vi "Begin.vi"(8 "error in":errorcluster) -> (0 "error out":errorcluster)   [LabVIEW 2020]
doc: "Called before other user functions, this VI is expected to open initial I/O refnums, load in file data, and do all program initialization. Notice that the <B>error out</B> terminal is simply used for data flow. Wiring it to other structures or subVIs ensures that this VI runs first."
uses:
  <vilib>/Rock Robotics/WPI/ThirdParty/Phoenix-LabVIEW/Pigeon2/controls/CTRE_Phoenix_Pigeon2_Configurables.ctl
  <vilib>/Rock Robotics/WPI/DriverStation/WPI_DriverStationRobotMode2.ctl
  <vilib>/Rock Robotics/SystemInterfaces/i2clib/i2c_bus.ctl
  <vilib>/Rock Robotics/WPI/Solenoid/WPI_SolenoidChannel.ctl
  <vilib>/Rock Robotics/SystemInterfaces/DIO/FPGA_DIOChannel.ctl
  <vilib>/Rock Robotics/WPI/Joystick/WPI_JoystickDeviceEnum.ctl
  Robot Global Data.vi
  <vilib>/Rock Robotics/WPI/Solenoid/WPI_SolenoidOpenDouble.vi
  <vilib>/Rock Robotics/WPI/Utilities/WPI_GetSetVariantRefNum.vi
  <vilib>/Rock Robotics/WPI/Switch/WPI_SwitchOpenCounting.vi
  <vilib>/Rock Robotics/WPI/Switch/WPI_SwitchOpenLimit.vi
  <vilib>/Rock Robotics/WPI/ThirdParty/Phoenix-LabVIEW/Motor Controller/Get/CTRE_Phoenix_MotorController_GetSelectedSensorData.vi
panel:
  in  "Pigeon2 Configurables":T1
  # "Yaw Angle needed to reach the current orientation in degrees"
  # "Configures the mounting pose of the Pigeon2\nThis is the yaw-pitch-roll teh Pigeon2 underwent to get to its current orientation,\n referenced from the robot's point of view\nThis is only necessary if the Pigeon2 is mounted at an exotic angle near the gimbal lock point or not forward.\nIf the pigeon is relatively flat and pointed forward, this is not needed"
  # "Pitch Angle needed to reach the current orientation in degrees"
  # "Roll Angle needed to reach the current orientation in degrees"
  # "Disables the temperature compensation\nfrom the Pigeon2. It is recommended that\nthis remains false"
  # "Disables the no-motion calibration from the\nPigeon2. It is recommended that this \nremains false"
  # "Enables the compass for Pigeon2\nThis is not recommended for any indoor robotics"
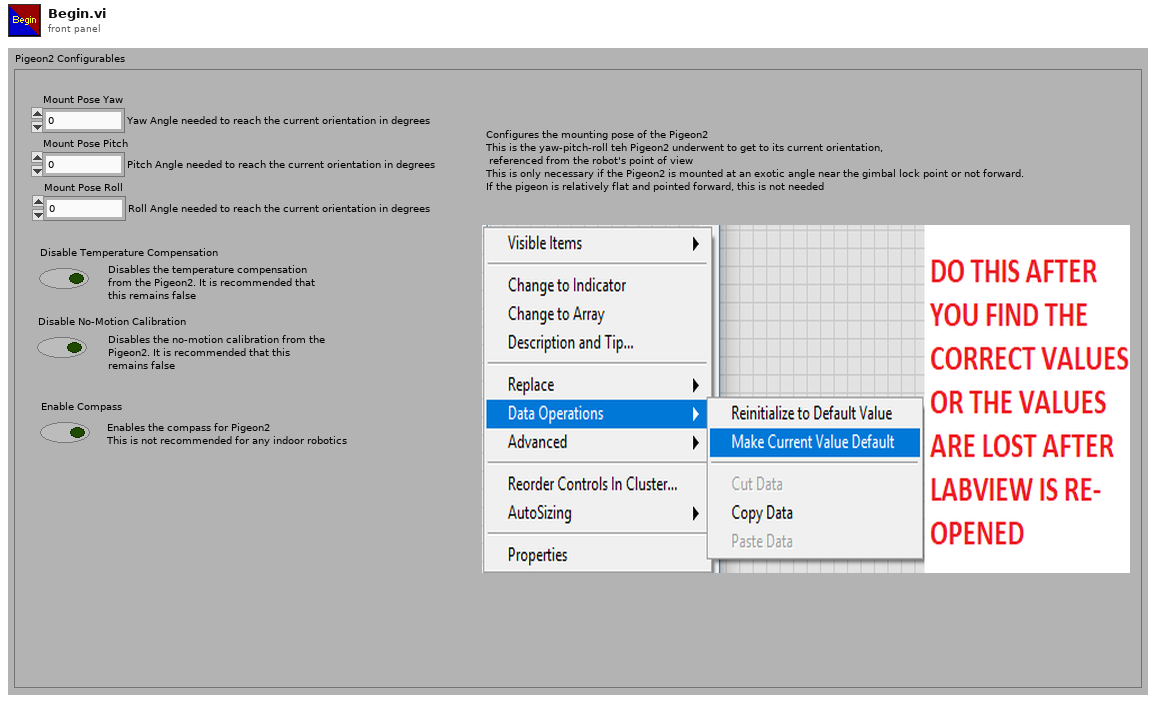
[diagram p1: front panel]
types:
  T1 = typedef "CTRE_Phoenix_Pigeon2_Configurables.ctl" = cluster{"Mount Pose Yaw":dbl, "Mount Pose Pitch":dbl, "Mount Pose Roll":dbl, "Disable Temperature Compensation":bool, "Disable No-Motion Calibration":bool, "Enable Compass":bool}
  T2 = typedef "FPGA_DIOChannel.ctl" = enum8{"DIO 0", "DIO 1", "DIO 2", "DIO 3", "DIO 4", "DIO 5", "DIO 6", "DIO 7", "DIO 8", "DIO 9", "DIO MXP 0", "DIO MXP 1", "DIO MXP 2", "DIO MXP 3", "DIO MXP 4", "DIO MXP 5", "DIO MXP 6", "DIO MXP 7", "DIO MXP 8", "DIO MXP 9", "DIO MXP 10", "DIO MXP 11", "DIO MXP 12", "DIO MXP 13", "DIO MXP 14", "DIO MXP 15", "SPI Port CS1", "SPI Port CS2", "SPI Port CS3", "SPI Port MISO", "SPI Port MOSI", "Invalid"}
  T3 = typedef "WPI_JoystickDeviceEnum.ctl" = enum16{"USB 0", "USB 1", "USB 2", "USB 3", "USB 4", "USB 5"}
  T4 = typedef "WPI_SolenoidChannel.ctl" = enum8{"Solenoid 0", "Solenoid 1", "Solenoid 2", "Solenoid 3", "Solenoid 4", "Solenoid 5", "Solenoid 6", "Solenoid 7", "Solenoid 8", "Solenoid 9", "Solenoid 10", "Solenoid 11", "Solenoid 12", "Solenoid 13", "Solenoid 14", "Solenoid 15", "Invalid"}
  T5 = typedef "i2c_bus.ctl" = enum16{"I2C On-Board", "I2C MXP", "Invalid"}
  T6 = typedef "WPI_DriverStationRobotMode2.ctl" = enum16{"Autonomous Disabled", "Autonomous Enabled", "Teleop Disabled", "Teleop Enabled", "Disconnected", "Finish", "Test Disabled", "Test Enabled", "Emergency Stopped"}
  T7 = typedef "WPI_JoystickDevRef.ctl" = cluster{"Device":T3}
  T8 = typedef "WPI_CompressorDevRef.ctl" = cluster{"DevStatus":errorcluster, "Pneumatics Control Module":u8}
  T9 = typedef "Color Sensor V3 DevRef.ctl" = cluster{"I2CDevRef":T10}
  T10 = typedef "WPI_I2CDevRef.ctl" = cluster{"DevStatus":errorcluster, "Device Address":u8, "Handle":i32, "I2C Bus":T5}
  T11 = typedef "WPI_SolenoidDevRef.ctl" = cluster{"DevStatus":errorcluster, "Pneumatics Control Module":u8, "Forward Solenoid Channel":T4, "Reverse Solenoid Channel":T4}
  T12 = typedef "WPI_MotorControlDeviceRef.ctl" = cluster{"DeviceStatus":errorcluster, "Type":T13, "PWM":cluster{"PWM Channel":T14, "DeadBand":T15}, "CAN":cluster{"Device Number":u8, "SetOutput VI Ref":variant, "GetOutput VI Ref":variant, "Enable VI Ref":variant, "Disable VI Ref":variant, "Data":variant}, "Invert":bool, "DIO PWM":cluster{"PWM \"Enable\" Channel":T14, "DIOChannel":T2, "PWM Rate":dbl}}
  T13 = typedef "WPI_MotorControlType.ctl" = enum16{"PWM", "CAN", "DIO PWM"}
  T14 = typedef "FPGA_DIOPWMChannel.ctl" = enum8{"PWM 0", "PWM 1", "PWM 2", "PWM 3", "PWM 4", "PWM 5", "PWM 6", "PWM 7", "PWM 8", "PWM 9", "PWM MXP 0", "PWM MXP 1", "PWM MXP 2", "PWM MXP 3", "PWM MXP 4", "PWM MXP 5", "PWM MXP 6", "PWM MXP 7", "PWM MXP 8", "PWM MXP 9", "Invalid"}
  T15 = typedef "WPI_PWMDeadband.ctl" = cluster{"Name":string, "maxPositivePwm":i32, "minPositivePwm":i32, "centerPwm":i32, "maxNegativePwm":i32, "minNegativePwm":i32, "angularRange":u16}
  T16 = typedef "CTRE_PigeonIMU_DeviceRef.ctl" = cluster{"DeviceStatus":errorcluster, "Device Number":u8, "Type":T17, "Device ID":u32, "Handle":u64, "UsageFrame":u32, "Library Path":path}
  T17 = typedef "CTRE_PigeonIMU_ConnectionType.ctl" = u32
  T18 = typedef "CTRE_Phoenix_CANcoder_DeviceRef.ctl" = cluster{"DeviceStatus":errorcluster, "Device Number":u8, "Handle":u64, "UsageFrame":u32, "Library Path":path}
  T19 = typedef "WPI_SwitchDevRef.ctl" = cluster{"DevStatus":errorcluster, "DIO Channel":T2, "CntIndex":T20, "Normally Closed":bool}
  T20 = typedef "FPGA_CounterCtrSystemIndex.ctl" = enum8{"Ctr 0", "Ctr 1", "Ctr 2", "Ctr 3", "Ctr 4", "Ctr 5", "Ctr 6", "Ctr 7", "Invalid"}
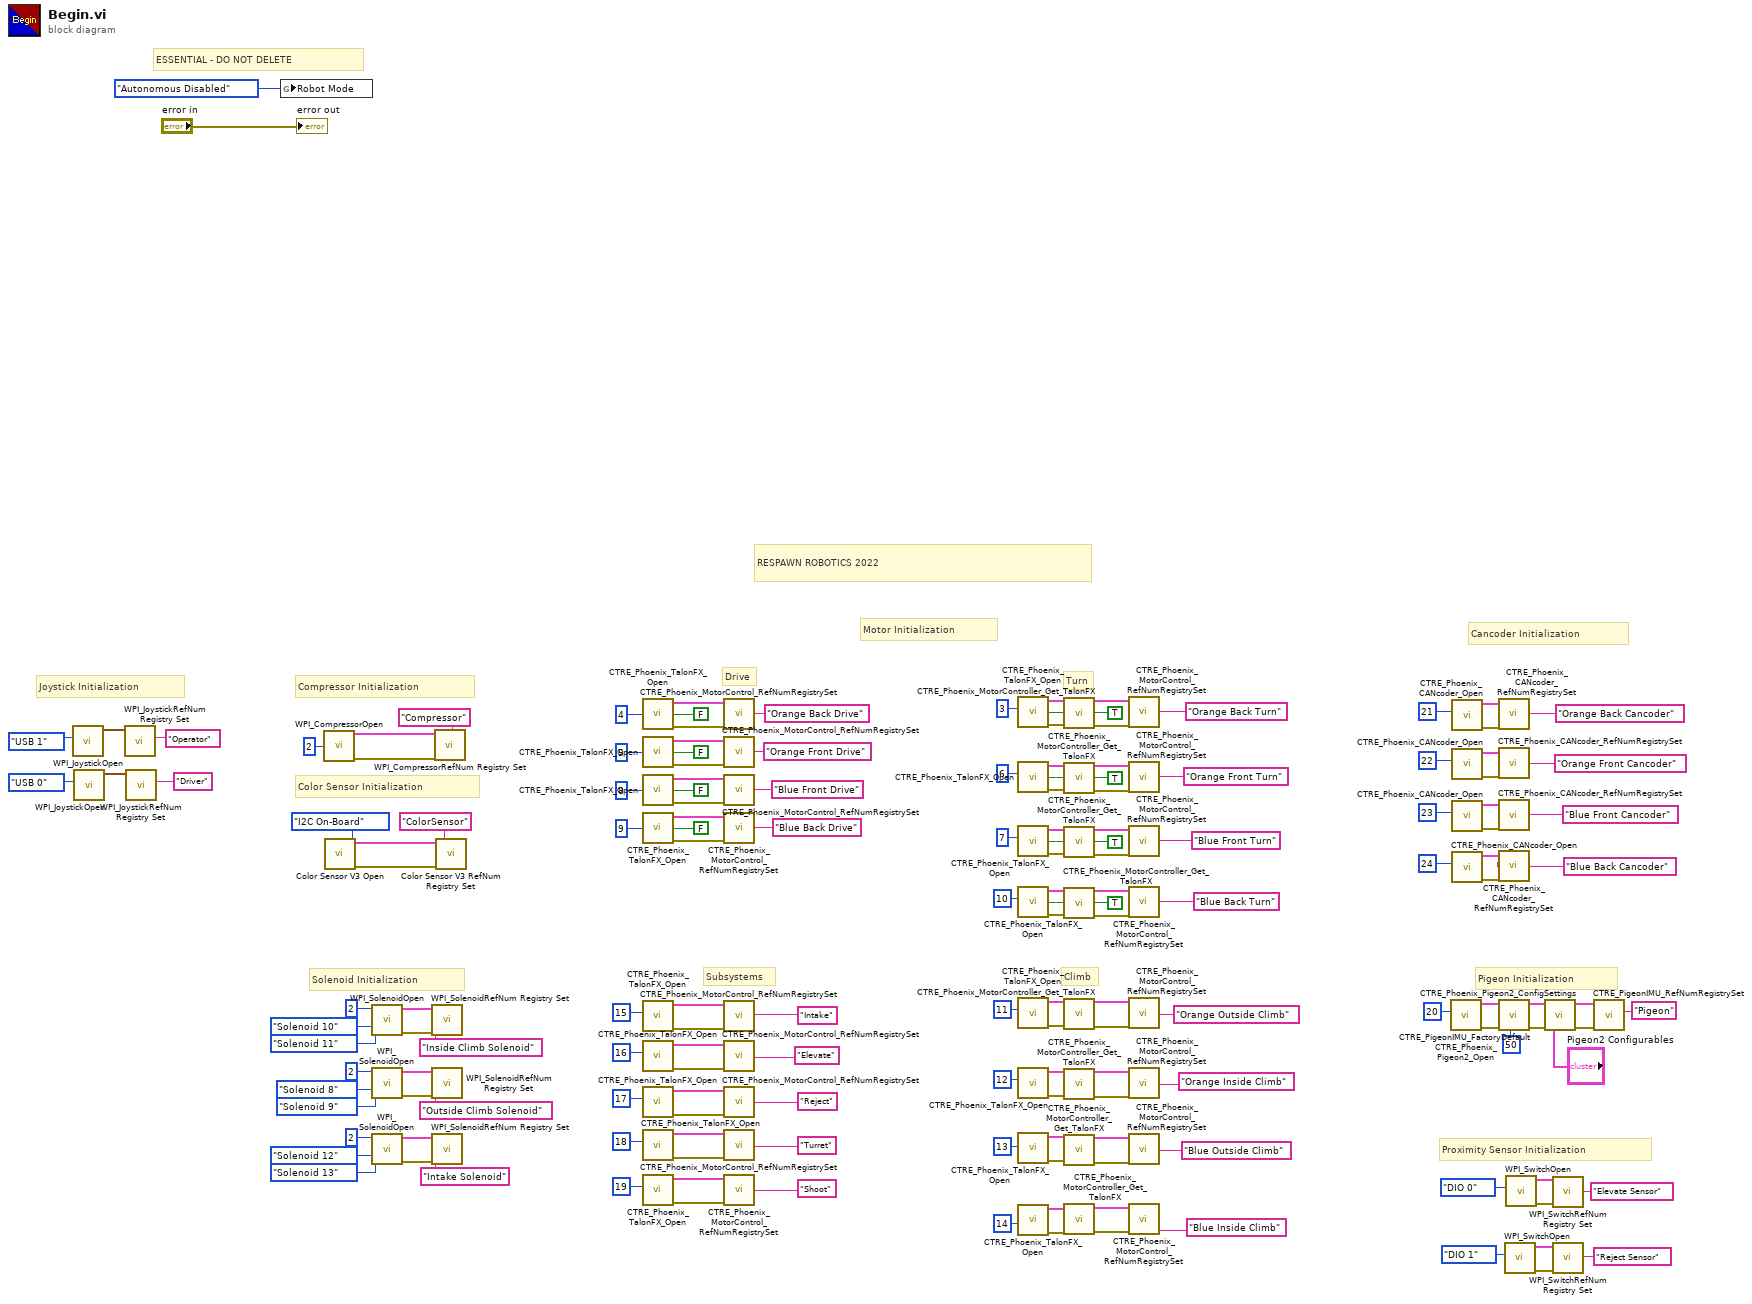
[diagram p0: block diagram]
diagram:
  # "Proximity Sensor Initialization"
  # "Pigeon Initialization"
  # "Cancoder Initialization"
  # "Solenoid Initialization"
  # "Color Sensor Initialization"
  # "Compressor Initialization"
  # "Climb"
  # "Subsystems"
  # "Turn"
  # "Drive"
  # "Motor Initialization"
  # "Joystick Initialization"
  # "RESPAWN ROBOTICS 2022"
  # "ESSENTIAL - DO NOT DELETE"
  n1 = call <vilib>:"WPI_JoystickOpen.vi"("JoystickDevice"=WPI_JoystickDeviceEnum."USB 1") -> ("JoystickDevRef"=w118:T7)  [unwired: 10 in]
  n2 = call <vilib>:"WPI_JoystickOpen.vi"("JoystickDevice"=WPI_JoystickDeviceEnum."USB 0") -> ("JoystickDevRef"=w121:T7)  [unwired: 10 in]
  n3 = call <vilib>:"WPI_JoystickRefNum Registry Set.vi"("refnum name"="Operator", "JoystickDevRef"=w118) -> ()  [unwired: 8 in, 2 out]
  n4 = call <vilib>:"WPI_JoystickRefNum Registry Set.vi"("refnum name"="Driver", "JoystickDevRef"=w121) -> ()  [unwired: 8 in, 2 out]
  n5 = global write "Robot Global Data.vi" "Robot Mode"(WPI_DriverStationRobotMode2."Autonomous Disabled" ("Robot Mode")) -> ()
  n6 = call <vilib>:"WPI_CompressorOpen.vi"("Pneumatics device (def)"=u8 2) -> ("CompressorDevRef"=w151:T8, "error out"=w152:errorcluster)  [unwired: 13 in]
  n7 = call <vilib>:"Color Sensor V3 Open.vi"("I2C Bus"=i2c_bus."I2C On-Board") -> ("error out"=w158:errorcluster, "ColorSensorDevRef"=w157:T9)  [unwired: 9 in]
  n8 = call-poly <vilib>:"WPI_SolenoidOpen.vi"("Reverse Solenoid Channel"=WPI_SolenoidChannel."Solenoid 11", "Forward Solenoid Channel"=WPI_SolenoidChannel."Solenoid 10", "Pneumatics Device (def)"=u8 2) -> ("error out"=w154:errorcluster, "SolenoidDevRef"=w153:T11)  [unwired: 7 in]
  n9 = call-poly <vilib>:"WPI_SolenoidOpen.vi"("Reverse Solenoid Channel"=WPI_SolenoidChannel."Solenoid 9", "Forward Solenoid Channel"=WPI_SolenoidChannel."Solenoid 8", "Pneumatics Device (def)"=u8 2) -> ("error out"=w140:errorcluster, "SolenoidDevRef"=w139:T11)  [unwired: 7 in]
  n10 = call-poly <vilib>:"WPI_SolenoidOpen.vi"("Reverse Solenoid Channel"=WPI_SolenoidChannel."Solenoid 13", "Forward Solenoid Channel"=WPI_SolenoidChannel."Solenoid 12", "Pneumatics Device (def)"=u8 2) -> ("error out"=w138:errorcluster, "SolenoidDevRef"=w137:T11)  [unwired: 7 in]
  n11 = call <vilib>:"WPI_SolenoidRefNum Registry Set.vi"("error in (no error)"=w154, "refnum name"="Inside Climb Solenoid", "SolenoidDevRef"=w153) -> ()  [unwired: 7 in, 2 out]
  n12 = call <vilib>:"WPI_SolenoidRefNum Registry Set.vi"("error in (no error)"=w140, "refnum name"="Outside Climb Solenoid", "SolenoidDevRef"=w139) -> ()  [unwired: 7 in, 2 out]
  n13 = call <vilib>:"WPI_SolenoidRefNum Registry Set.vi"("error in (no error)"=w138, "refnum name"="Intake Solenoid", "SolenoidDevRef"=w137) -> ()  [unwired: 7 in, 2 out]
  n14 = call <vilib>:"WPI_CompressorRefNum Registry Set.vi"("error in (no error)"=w152, "refnum name"="Compressor", "CompressorDevRef"=w151) -> ()  [unwired: 7 in, 2 out]
  n15 = call <vilib>:"Color Sensor V3 RefNum Registry Set.vi"("error in (no error)"=w158, "refnum name"="ColorSensor", "ColorSensorDevRef"=w157) -> ()  [unwired: 7 in, 2 out]
  n16 = call <vilib>:"CTRE_Phoenix_TalonFX_Open.vi"("Invert"=FALSE, "Device Number"=u8 4) -> ("error out"=w116:errorcluster, "PhoenixMotorControlDevRef"=w115:T12)  [unwired: 8 in]
  n17 = call <vilib>:"CTRE_Phoenix_TalonFX_Open.vi"("Invert"=FALSE, "Device Number"=u8 5) -> ("error out"=w111:errorcluster, "PhoenixMotorControlDevRef"=w110:T12)  [unwired: 8 in]
  n18 = call <vilib>:"CTRE_Phoenix_TalonFX_Open.vi"("Invert"=FALSE, "Device Number"=u8 8) -> ("error out"=w106:errorcluster, "PhoenixMotorControlDevRef"=w105:T12)  [unwired: 8 in]
  n19 = call <vilib>:"CTRE_Phoenix_TalonFX_Open.vi"("Invert"=FALSE, "Device Number"=u8 9) -> ("error out"=w101:errorcluster, "PhoenixMotorControlDevRef"=w100:T12)  [unwired: 8 in]
  n20 = call <vilib>:"CTRE_Phoenix_TalonFX_Open.vi"("Device Number"=u8 15) -> ("error out"=w64:errorcluster, "PhoenixMotorControlDevRef"=w63:T12)  [unwired: 9 in]
  n21 = call <vilib>:"CTRE_Phoenix_TalonFX_Open.vi"("Device Number"=u8 16) -> ("error out"=w68:errorcluster, "PhoenixMotorControlDevRef"=w67:T12)  [unwired: 9 in]
  n22 = call <vilib>:"CTRE_Phoenix_TalonFX_Open.vi"("Device Number"=u8 17) -> ("error out"=w60:errorcluster, "PhoenixMotorControlDevRef"=w59:T12)  [unwired: 9 in]
  n23 = call <vilib>:"CTRE_Phoenix_TalonFX_Open.vi"("Device Number"=u8 18) -> ("error out"=w52:errorcluster, "PhoenixMotorControlDevRef"=w51:T12)  [unwired: 9 in]
  n24 = call <vilib>:"CTRE_Phoenix_TalonFX_Open.vi"("Device Number"=u8 19) -> ("error out"=w56:errorcluster, "PhoenixMotorControlDevRef"=w55:T12)  [unwired: 9 in]
  n25 = call <vilib>:"CTRE_Phoenix_MotorControl_RefNumRegistrySet.vi"("error in (no error)"=w116, "refnum name"="Orange Back Drive", "PhoenixMotorControlDevRef"=w115) -> ()  [unwired: 7 in, 2 out]
  n26 = call <vilib>:"CTRE_Phoenix_MotorControl_RefNumRegistrySet.vi"("error in (no error)"=w111, "refnum name"="Orange Front Drive", "PhoenixMotorControlDevRef"=w110) -> ()  [unwired: 7 in, 2 out]
  n27 = call <vilib>:"CTRE_Phoenix_MotorControl_RefNumRegistrySet.vi"("error in (no error)"=w106, "refnum name"="Blue Front Drive", "PhoenixMotorControlDevRef"=w105) -> ()  [unwired: 7 in, 2 out]
  n28 = call <vilib>:"CTRE_Phoenix_MotorControl_RefNumRegistrySet.vi"("error in (no error)"=w101, "refnum name"="Blue Back Drive", "PhoenixMotorControlDevRef"=w100) -> ()  [unwired: 7 in, 2 out]
  n29 = call <vilib>:"CTRE_Phoenix_MotorControl_RefNumRegistrySet.vi"("error in (no error)"=w64, "refnum name"="Intake", "PhoenixMotorControlDevRef"=w63) -> ()  [unwired: 7 in, 2 out]
  n30 = call <vilib>:"CTRE_Phoenix_MotorControl_RefNumRegistrySet.vi"("error in (no error)"=w68, "refnum name"="Elevate", "PhoenixMotorControlDevRef"=w67) -> ()  [unwired: 7 in, 2 out]
  n31 = call <vilib>:"CTRE_Phoenix_MotorControl_RefNumRegistrySet.vi"("error in (no error)"=w60, "refnum name"="Reject", "PhoenixMotorControlDevRef"=w59) -> ()  [unwired: 7 in, 2 out]
  n32 = call <vilib>:"CTRE_Phoenix_MotorControl_RefNumRegistrySet.vi"("error in (no error)"=w52, "refnum name"="Turret", "PhoenixMotorControlDevRef"=w51) -> ()  [unwired: 7 in, 2 out]
  n33 = call <vilib>:"CTRE_Phoenix_MotorControl_RefNumRegistrySet.vi"("error in (no error)"=w56, "refnum name"="Shoot", "PhoenixMotorControlDevRef"=w55) -> ()  [unwired: 7 in, 2 out]
  n34 = call <vilib>:"CTRE_Phoenix_TalonFX_Open.vi"("Invert"=TRUE, "Device Number"=u8 3) -> ("error out"=w95:errorcluster, "PhoenixMotorControlDevRef"=w96:T12)  [unwired: 8 in]
  n35 = call <vilib>:"CTRE_Phoenix_TalonFX_Open.vi"("Invert"=TRUE, "Device Number"=u8 6) -> ("error out"=w88:errorcluster, "PhoenixMotorControlDevRef"=w89:T12)  [unwired: 8 in]
  n36 = call <vilib>:"CTRE_Phoenix_TalonFX_Open.vi"("Invert"=TRUE, "Device Number"=u8 7) -> ("error out"=w81:errorcluster, "PhoenixMotorControlDevRef"=w82:T12)  [unwired: 8 in]
  n37 = call <vilib>:"CTRE_Phoenix_TalonFX_Open.vi"("Invert"=TRUE, "Device Number"=u8 10) -> ("error out"=w74:errorcluster, "PhoenixMotorControlDevRef"=w75:T12)  [unwired: 8 in]
  n38 = call <vilib>:"CTRE_Phoenix_TalonFX_Open.vi"("Device Number"=u8 11) -> ("error out"=w47:errorcluster, "PhoenixMotorControlDevRef"=w48:T12)  [unwired: 9 in]
  n39 = call <vilib>:"CTRE_Phoenix_TalonFX_Open.vi"("Device Number"=u8 12) -> ("error out"=w41:errorcluster, "PhoenixMotorControlDevRef"=w42:T12)  [unwired: 9 in]
  n40 = call <vilib>:"CTRE_Phoenix_TalonFX_Open.vi"("Device Number"=u8 13) -> ("error out"=w35:errorcluster, "PhoenixMotorControlDevRef"=w36:T12)  [unwired: 9 in]
  n41 = call <vilib>:"CTRE_Phoenix_TalonFX_Open.vi"("Device Number"=u8 14) -> ("error out"=w29:errorcluster, "PhoenixMotorControlDevRef"=w30:T12)  [unwired: 9 in]
  n42 = call-poly <vilib>:"CTRE_Phoenix_MotorController_Get_TalonFX.vi"("PhoenixMotorControlDevRef"=w96, "error in"=w95) -> ("PhoenixMotorControlDevRef"=w93:T12, "error out"=w94:errorcluster)  [unwired: 10 in, 2 out]
  n43 = call-poly <vilib>:"CTRE_Phoenix_MotorController_Get_TalonFX.vi"("PhoenixMotorControlDevRef"=w89, "error in"=w88) -> ("PhoenixMotorControlDevRef"=w86:T12, "error out"=w87:errorcluster)  [unwired: 10 in, 2 out]
  n44 = call-poly <vilib>:"CTRE_Phoenix_MotorController_Get_TalonFX.vi"("PhoenixMotorControlDevRef"=w82, "error in"=w81) -> ("PhoenixMotorControlDevRef"=w79:T12, "error out"=w80:errorcluster)  [unwired: 10 in, 2 out]
  n45 = call-poly <vilib>:"CTRE_Phoenix_MotorController_Get_TalonFX.vi"("PhoenixMotorControlDevRef"=w75, "error in"=w74) -> ("PhoenixMotorControlDevRef"=w72:T12, "error out"=w73:errorcluster)  [unwired: 10 in, 2 out]
  n46 = call-poly <vilib>:"CTRE_Phoenix_MotorController_Get_TalonFX.vi"("PhoenixMotorControlDevRef"=w48, "error in"=w47) -> ("PhoenixMotorControlDevRef"=w45:T12, "error out"=w46:errorcluster)  [unwired: 10 in, 2 out]
  n47 = call-poly <vilib>:"CTRE_Phoenix_MotorController_Get_TalonFX.vi"("PhoenixMotorControlDevRef"=w42, "error in"=w41) -> ("PhoenixMotorControlDevRef"=w39:T12, "error out"=w40:errorcluster)  [unwired: 10 in, 2 out]
  n48 = call-poly <vilib>:"CTRE_Phoenix_MotorController_Get_TalonFX.vi"("PhoenixMotorControlDevRef"=w36, "error in"=w35) -> ("PhoenixMotorControlDevRef"=w33:T12, "error out"=w34:errorcluster)  [unwired: 10 in, 2 out]
  n49 = call-poly <vilib>:"CTRE_Phoenix_MotorController_Get_TalonFX.vi"("PhoenixMotorControlDevRef"=w30, "error in"=w29) -> ("PhoenixMotorControlDevRef"=w25:T12, "error out"=w28:errorcluster)  [unwired: 10 in, 2 out]
  n50 = call <vilib>:"CTRE_Phoenix_MotorControl_RefNumRegistrySet.vi"("error in (no error)"=w94, "refnum name"="Orange Back Turn", "PhoenixMotorControlDevRef"=w93) -> ()  [unwired: 7 in, 2 out]
  n51 = call <vilib>:"CTRE_Phoenix_MotorControl_RefNumRegistrySet.vi"("error in (no error)"=w87, "refnum name"="Orange Front Turn", "PhoenixMotorControlDevRef"=w86) -> ()  [unwired: 7 in, 2 out]
  n52 = call <vilib>:"CTRE_Phoenix_MotorControl_RefNumRegistrySet.vi"("error in (no error)"=w80, "refnum name"="Blue Front Turn", "PhoenixMotorControlDevRef"=w79) -> ()  [unwired: 7 in, 2 out]
  n53 = call <vilib>:"CTRE_Phoenix_MotorControl_RefNumRegistrySet.vi"("error in (no error)"=w73, "refnum name"="Blue Back Turn", "PhoenixMotorControlDevRef"=w72) -> ()  [unwired: 7 in, 2 out]
  n54 = call <vilib>:"CTRE_Phoenix_MotorControl_RefNumRegistrySet.vi"("error in (no error)"=w46, "refnum name"="Orange Outside Climb", "PhoenixMotorControlDevRef"=w45) -> ()  [unwired: 7 in, 2 out]
  n55 = call <vilib>:"CTRE_Phoenix_MotorControl_RefNumRegistrySet.vi"("error in (no error)"=w40, "refnum name"="Orange Inside Climb", "PhoenixMotorControlDevRef"=w39) -> ()  [unwired: 7 in, 2 out]
  n56 = call <vilib>:"CTRE_Phoenix_MotorControl_RefNumRegistrySet.vi"("error in (no error)"=w34, "refnum name"="Blue Outside Climb", "PhoenixMotorControlDevRef"=w33) -> ()  [unwired: 7 in, 2 out]
  n57 = call <vilib>:"CTRE_Phoenix_MotorControl_RefNumRegistrySet.vi"("error in (no error)"=w28, "refnum name"="Blue Inside Climb", "PhoenixMotorControlDevRef"=w25) -> ()  [unwired: 7 in, 2 out]
  n58 = call <vilib>:"CTRE_Phoenix_Pigeon2_Open.vi"("Device Number"=u8 20) -> ("error out"=w150:errorcluster, "PigeonIMUDevRef"=w149:T16)  [unwired: 9 in]
  n59 = call <vilib>:"CTRE_Phoenix_CANcoder_Open.vi"("Device Number"=u8 21) -> ("error out"=w24:errorcluster, "CTRE_CANcoder_DeviceRef"=w23:T18)  [unwired: 9 in]
  n60 = call <vilib>:"CTRE_Phoenix_CANcoder_Open.vi"("Device Number"=u8 22) -> ("error out"=w20:errorcluster, "CTRE_CANcoder_DeviceRef"=w19:T18)  [unwired: 9 in]
  n61 = call <vilib>:"CTRE_Phoenix_CANcoder_Open.vi"("Device Number"=u8 23) -> ("error out"=w16:errorcluster, "CTRE_CANcoder_DeviceRef"=w15:T18)  [unwired: 9 in]
  n62 = call <vilib>:"CTRE_Phoenix_CANcoder_Open.vi"("Device Number"=u8 24) -> ("error out"=w12:errorcluster, "CTRE_CANcoder_DeviceRef"=w11:T18)  [unwired: 9 in]
  n63 = call <vilib>:"CTRE_Phoenix_CANcoder_RefNumRegistrySet.vi"("error in (no error)"=w24, "refnum name"="Orange Back Cancoder", "CTRE_CANcoder_DeviceRef"=w23) -> ()  [unwired: 7 in, 2 out]
  n64 = call <vilib>:"CTRE_Phoenix_CANcoder_RefNumRegistrySet.vi"("error in (no error)"=w20, "refnum name"="Orange Front Cancoder", "CTRE_CANcoder_DeviceRef"=w19) -> ()  [unwired: 7 in, 2 out]
  n65 = call <vilib>:"CTRE_Phoenix_CANcoder_RefNumRegistrySet.vi"("error in (no error)"=w16, "refnum name"="Blue Front Cancoder", "CTRE_CANcoder_DeviceRef"=w15) -> ()  [unwired: 7 in, 2 out]
  n66 = call <vilib>:"CTRE_Phoenix_CANcoder_RefNumRegistrySet.vi"("error in (no error)"=w12, "refnum name"="Blue Back Cancoder", "CTRE_CANcoder_DeviceRef"=w11) -> ()  [unwired: 7 in, 2 out]
  n67 = call <vilib>:"CTRE_PigeonIMU_FactoryDefault.vi"("timeoutMs"=50, "error in"=w150, "PigeonIMUDevRef"=w149) -> ("error out"=w148:errorcluster, "PigeonIMUDevRef"=w147:T16)  [unwired: 7 in]
  n68 = call-poly <vilib>:"WPI_SwitchOpen.vi"("DIO Channel"=FPGA_DIOChannel."DIO 1") -> ("error out"=w5:errorcluster, "SwitchDevRef"=w6:T19)  [unwired: 9 in]
  n69 = call-poly <vilib>:"WPI_SwitchOpen.vi"("DIO Channel"=FPGA_DIOChannel."DIO 0") -> ("error out"=w1:errorcluster, "SwitchDevRef"=w2:T19)  [unwired: 9 in]
  n70 = call <vilib>:"CTRE_Phoenix_Pigeon2_ConfigSettings.vi"("error in (no error)"=w148, "Pigeon2 Configurables"="Pigeon2 Configurables", "PigeonIMUDevRef 2"=w147) -> ("error out"=w146:errorcluster, "PigeonIMUDevRef"=w145:T16)  [unwired: 7 in]
  n71 = call <vilib>:"WPI_SwitchRefNum Registry Set.vi"("error in (no error)"=w1, "refnum name"="Elevate Sensor", "SwitchDevRef"=w2) -> ()  [unwired: 7 in, 2 out]
  n72 = call <vilib>:"WPI_SwitchRefNum Registry Set.vi"("error in (no error)"=w5, "refnum name"="Reject Sensor", "SwitchDevRef"=w6) -> ()  [unwired: 7 in, 2 out]
  n73 = call <vilib>:"CTRE_PigeonIMU_RefNumRegistrySet.vi"("error in (no error)"=w146, "refnum name"="Pigeon", "PigeonIMUDevRef"=w145) -> ()  [unwired: 7 in, 2 out]
  "error out" <- "error in"
